vi "ValidateTiming.vi"(8 "Error In":errorcluster, 11 "MasterCluster In":T1={"Plate Reader State"=enum."Idle", "SMPAutomationClientRef"=refnum, "CommandCompleted Refnum"=refnum, "InstrumentStatusChanged Refnum"=refnum, "ErrorReport Refnum"=refnum, "Read Start Time"=timestamp(0 s since 1904-01-01), "Read Count"=0, "Active Column"=0, "Raw Result"="", "GetDataCopy CMD Queue ID"=0, "Error Log"="", "Column Data"={"Col Absorbances"=[], "Col Read Times"=[], "Col Read Positions (deg)"=[], "Temperature (degC)"=0.0, "Active Column"=0, "Previous Column"=0, "Column Read Start Time"=timestamp(0 s since 1904-01-01), "Column Busy Start Time"=timestamp(0 s since 1904-01-01), "Column Busy Stop Time"=timestamp(0 s since 1904-01-01), "Column Mark Read Start Time"=timestamp(0 s since 1904-01-01), "Column Mark Read Stop Time"=timestamp(0 s since 1904-01-01)}, "Grid"=[[0.0, 0.0, 0.0, 0.0, 0.0, 0.0, 0.0, 0.0, 0.0, 0.0, 0.0, 0.0], [0.0, 0.0, 0.0, 0.0, 0.0, 0.0, 0.0, 0.0, 0.0, 0.0, 0.0, 0.0], [0.0, 0.0, 0.0, 0.0, 0.0, 0.0, 0.0, 0.0, 0.0, 0.0, 0.0, 0.0], [0.0, 0.0, 0.0, 0.0, 0.0, 0.0, 0.0, 0.0, 0.0, 0.0, 0.0, 0.0], [0.0, 0.0, 0.0, 0.0, 0.0, 0.0, 0.0, 0.0, 0.0, 0.0, 0.0, 0.0], [0.0, 0.0, 0.0, 0.0, 0.0, 0.0, 0.0, 0.0, 0.0, 0.0, 0.0, 0.0], [0.0, 0.0, 0.0, 0.0, 0.0, 0.0, 0.0, 0.0, 0.0, 0.0, 0.0, 0.0], [0.0, 0.0, 0.0, 0.0, 0.0, 0.0, 0.0, 0.0, 0.0, 0.0, 0.0, 0.0]], "Column Read Start Time"=timestamp(0 s since 1904-01-01), "Previous Column"=0, "Raw Log File Refnum"=refnum, "Read Specifications"={"Read Period (min)"=0.0, "Experiment Duration (min)"=0.0, "Number of Columns"=0, "Apex Deviance (deg)"=0.0, "Log File Name"="", "Number of Wavelengths"=0, "Timing Profile"=enum."No Timing", "Column Switch Delay"=0.0, "Column Repeat Delay"=0.0, "Audible Read Delay"=0.0, "Audible Read Interval"=0.0, "SMP Protocol Path"=path "", "Upper Busy Delay Limit"=inf, "Lower Busy Delay Limit"=-inf, "Upper Busy Interval Limit"=inf, "Lower Busy Interval Limit"=-inf, "Number of Rows"=0, "Plate Reader COM Port"=""}, "Plate Reader Crash State"=enum."Idle", "Consecutive Missed Reads"=0, "Excel File Refnum"=refnum} {"Column Data"."Column Mark Read Stop Time" format="%<%H:%M:%S%3u\n%x>T"; "Column Data"."Column Mark Read Start Time" format="%<%H:%M:%S%3u\n%x>T"; "Column Data"."Column Busy Stop Time" format="%<%H:%M:%S%3u\n%x>T"; "Column Data"."Column Busy Start Time" format="%<%H:%M:%S%3u\n%x>T"; "Column Data"."Column Read Start Time" format="%<%H:%M:%S%3u\n%x>T"; "Column Data"."Col Read Times" format="%<%H:%M:%S%3u\n%x>T"}) -> (0 "Error Out":errorcluster, 3 "MasterCluster Out":T1={"Plate Reader State"=enum."Idle", "SMPAutomationClientRef"=refnum, "CommandCompleted Refnum"=refnum, "InstrumentStatusChanged Refnum"=refnum, "ErrorReport Refnum"=refnum, "Read Start Time"=timestamp(0 s since 1904-01-01), "Read Count"=0, "Active Column"=0, "Raw Result"="", "GetDataCopy CMD Queue ID"=0, "Error Log"="", "Column Data"={"Col Absorbances"=[], "Col Read Times"=[], "Col Read Positions (deg)"=[], "Temperature (degC)"=0.0, "Active Column"=0, "Previous Column"=0, "Column Read Start Time"=timestamp(0 s since 1904-01-01), "Column Busy Start Time"=timestamp(0 s since 1904-01-01), "Column Busy Stop Time"=timestamp(0 s since 1904-01-01), "Column Mark Read Start Time"=timestamp(0 s since 1904-01-01), "Column Mark Read Stop Time"=timestamp(0 s since 1904-01-01)}, "Grid"=[[0.0, 0.0, 0.0, 0.0, 0.0, 0.0, 0.0, 0.0, 0.0, 0.0, 0.0, 0.0], [0.0, 0.0, 0.0, 0.0, 0.0, 0.0, 0.0, 0.0, 0.0, 0.0, 0.0, 0.0], [0.0, 0.0, 0.0, 0.0, 0.0, 0.0, 0.0, 0.0, 0.0, 0.0, 0.0, 0.0], [0.0, 0.0, 0.0, 0.0, 0.0, 0.0, 0.0, 0.0, 0.0, 0.0, 0.0, 0.0], [0.0, 0.0, 0.0, 0.0, 0.0, 0.0, 0.0, 0.0, 0.0, 0.0, 0.0, 0.0], [0.0, 0.0, 0.0, 0.0, 0.0, 0.0, 0.0, 0.0, 0.0, 0.0, 0.0, 0.0], [0.0, 0.0, 0.0, 0.0, 0.0, 0.0, 0.0, 0.0, 0.0, 0.0, 0.0, 0.0], [0.0, 0.0, 0.0, 0.0, 0.0, 0.0, 0.0, 0.0, 0.0, 0.0, 0.0, 0.0]], "Column Read Start Time"=timestamp(0 s since 1904-01-01), "Previous Column"=0, "Raw Log File Refnum"=refnum, "Read Specifications"={"Read Period (min)"=0.0, "Experiment Duration (min)"=0.0, "Number of Columns"=0, "Apex Deviance (deg)"=0.0, "Log File Name"="", "Number of Wavelengths"=0, "Timing Profile"=enum."No Timing", "Column Switch Delay"=0.0, "Column Repeat Delay"=0.0, "Audible Read Delay"=0.0, "Audible Read Interval"=0.0, "SMP Protocol Path"=path "", "Upper Busy Delay Limit"=inf, "Lower Busy Delay Limit"=-inf, "Upper Busy Interval Limit"=inf, "Lower Busy Interval Limit"=-inf, "Number of Rows"=0, "Plate Reader COM Port"=""}, "Plate Reader Crash State"=enum."Idle", "Consecutive Missed Reads"=0, "Excel File Refnum"=refnum} {"Column Data"."Column Mark Read Stop Time" format="%<%H:%M:%S%3u\n%x>T"; "Column Data"."Column Mark Read Start Time" format="%<%H:%M:%S%3u\n%x>T"; "Column Data"."Column Busy Stop Time" format="%<%H:%M:%S%3u\n%x>T"; "Column Data"."Column Busy Start Time" format="%<%H:%M:%S%3u\n%x>T"; "Column Data"."Column Read Start Time" format="%<%H:%M:%S%3u\n%x>T"; "Column Data"."Col Read Times" format="%<%H:%M:%S%3u\n%x>T"})   [LabVIEW 2014]
uses:
  MasterCluster.ctl
  PlateReaderState.ctl
  C:/Program Files (x86)/Molecular Devices/SoftMax Pro 6.5.1 Automation SDK/SoftMaxPro.AutomationClient.dll
  Program Files (x86)/Molecular Devices/SoftMax Pro 6.5.1 Automation SDK/SoftMaxPro.AutomationClient.dll
  ColumnData.ctl
  ReadSpecifications.ctl
  TimingProfile.ctl
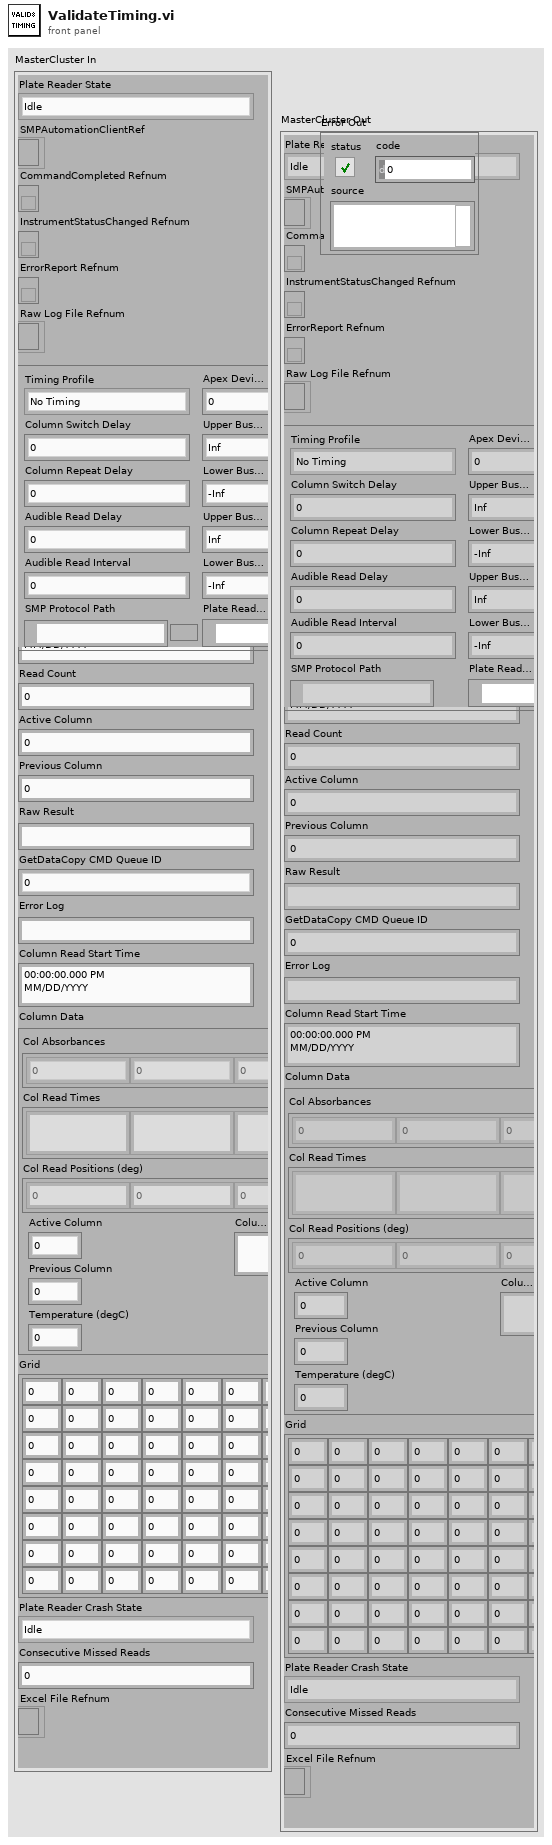
[diagram p1: front panel]
types:
  T1 = typedef "MasterCluster.ctl" = cluster{"Plate Reader State":T2, "SMPAutomationClientRef":refnum<k24>, "CommandCompleted Refnum":refnum<k27>, "InstrumentStatusChanged Refnum":refnum<k27>, "ErrorReport Refnum":refnum<k27>, "Read Start Time":timestamp, "Read Count":u64, "Active Column":u64, "Raw Result":string, "GetDataCopy CMD Queue ID":i32, "Error Log":string, "Column Data":T3, "Grid":dbl[][], "Column Read Start Time":timestamp, "Previous Column":u64, "Raw Log File Refnum":refnum<file>, "Read Specifications":T4, "Plate Reader Crash State":T2, "Consecutive Missed Reads":u64, "Excel File Refnum":refnum<file>}
  T2 = typedef "PlateReaderState.ctl" = enum16{"Idle", "Run", "Wait", "Read", "Init", "Exit", "Stop"}
  T3 = typedef "ColumnData.ctl" = cluster{"Col Absorbances":dbl[], "Col Read Times":timestamp[], "Col Read Positions (deg)":dbl[], "Temperature (degC)":dbl, "Active Column":u64, "Previous Column":u64, "Column Read Start Time":timestamp, "Column Busy Start Time":timestamp, "Column Busy Stop Time":timestamp, "Column Mark Read Start Time":timestamp, "Column Mark Read Stop Time":timestamp}
  T4 = typedef "ReadSpecifications.ctl" = cluster{"Read Period (min)":dbl, "Experiment Duration (min)":dbl, "Number of Columns":u64, "Apex Deviance (deg)":dbl, "Log File Name":string, "Number of Wavelengths":u64, "Timing Profile":T5, "Column Switch Delay":dbl, "Column Repeat Delay":dbl, "Audible Read Delay":dbl, "Audible Read Interval":dbl, "SMP Protocol Path":path, "Upper Busy Delay Limit":dbl, "Lower Busy Delay Limit":dbl, "Upper Busy Interval Limit":dbl, "Lower Busy Interval Limit":dbl, "Number of Rows":u64, "Plate Reader COM Port":refnum<visa-resource-name>}
  T5 = typedef "TimingProfile.ctl" = enum16{"No Timing", "24-Well Fluorescence", "48-Well Fluorescence", "96-Well Fluorescence", "96-Well Absorbance", "Custom Timing"}
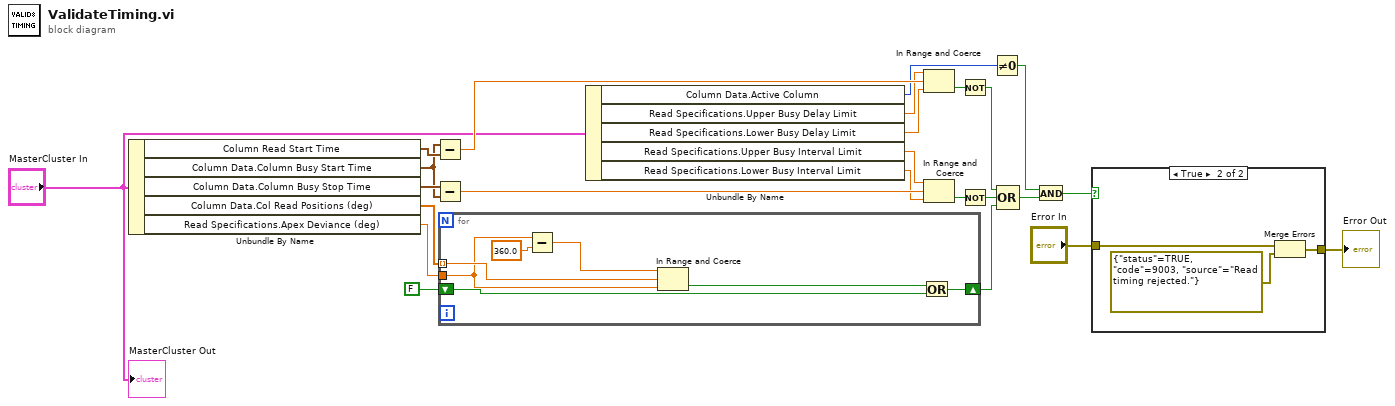
[diagram p0: block diagram]
diagram:
  n1 = Unbundle By Name("MasterCluster In") -> ("Column Read Start Time"=w21:timestamp, "Column Data.Column Busy Start Time"=w19:timestamp, "Column Data.Column Busy Stop Time"=w20:timestamp, "Column Data.Col Read Positions (deg)"=w24:dbl[], "Read Specifications.Apex Deviance (deg)"=w5:dbl)
  n2 = Subtract(x=w19, y=w21) -> (x-y=w18:dbl)
  n3 = Subtract(x=w20, y=w19) -> (x-y=w17:dbl)
  n4 = for {
    tunnel: w24 -> [w31] mode=indexing
    shift-right: [w26] -> w22
    shift-left: FALSE -> [w27]
    tunnel: w5 -> [w25]
    n5 = Subtract(x=w25, y=360.0) -> (x-y=w29:dbl)
    n6 = In Range and Coerce(upper limit=w29, x=w31, lower limit=w25) -> (In Range?=w28:bool)  [unwired: 1 out]
    n7 = Or(x=w28, y=w27) -> (x .or. y?=w26:bool)
  }
  n8 = Unbundle By Name("MasterCluster In") -> ("Column Data.Active Column"=w3:u64, "Read Specifications.Upper Busy Delay Limit"=w10:dbl, "Read Specifications.Lower Busy Delay Limit"=w9:dbl, "Read Specifications.Upper Busy Interval Limit"=w8:dbl, "Read Specifications.Lower Busy Interval Limit"=w7:dbl)
  n9 = In Range and Coerce(upper limit=w10, x=w18, lower limit=w9) -> (In Range?=w14:bool)  [unwired: 1 out]
  n10 = In Range and Coerce(upper limit=w8, x=w17, lower limit=w7) -> (In Range?=w13:bool)  [unwired: 1 out]
  n11 = Not(x=w14) -> (.not. x?=w11:bool)
  n12 = Not(x=w13) -> (.not. x?=w12:bool)
  n13 = Not Equal To 0?(x=w3) -> (x != 0?=w2:bool)
  n14 = Compound Arithmetic op=OR(w11, w12, w22) -> (w4:bool)
  n15 = And(x=w2, y=w4) -> (x .and. y?=w1:bool)
  n16 = case shown="True" w1 {
    tunnel: "Error In" -> [w32 w35]
    tunnel: [w32 w34] -> w15
    frame False {
    }
    frame True {
      n17 = Merge Errors(w35, errorcluster {"status"=TRUE, "code"=9003, "source"="Read timing rejected."} ("error in")) -> (w34:errorcluster)
    }
  }
  "Error Out" <- w15
  "MasterCluster Out" <- "MasterCluster In"
